vi "read_status_flash.vi"() -> ()   [LabVIEW 2022 SP3]
panel:
  out "InputReport1":u8[](array[numeric]) format="%x"
  out "Output Report":u8[](array[numeric])
  out "Input Report":u8[](array[numeric])
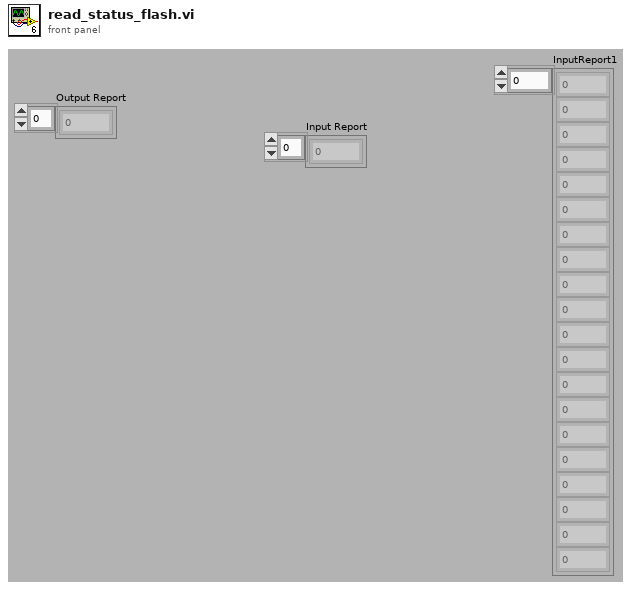
[diagram p1: front panel]
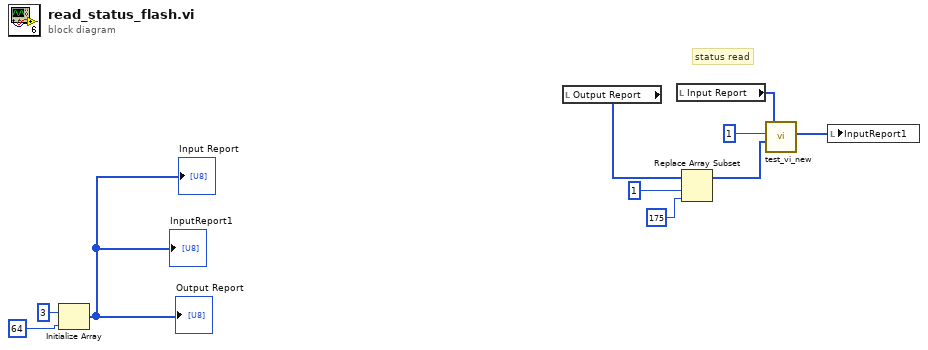
[diagram p0: block diagram]
diagram:
  # "status read"
  n1 = Initialize Array(u8 3 ("element"), 64 ("dimension size")) -> (→"Input Report" →"Output Report" →"InputReport1":u8[])
  n2 = local read "Output Report"() -> (w7:u8[])
  n3 = local read "Input Report"() -> (w6:u8[])
  n4 = Replace Array Subset(array=w7, new element=u8 175 ("new element/subarray"), index=1) -> (w5:u8[])
  n5 = call "test_vi_new.vi"("OutputReport_in"=w5, "DevDet_in"=1, "InputReport_in"=w6) -> ("InputReport_out"=w4:u8[])  [unwired: 1 in, 3 out]
  n6 = local write "InputReport1"(w4) -> ()
